vi "Actor Core.vi"(8 "error in":errorcluster, 11 "DAQ in":refnum<class "DAQ.lvclass">) -> (0 "error out":errorcluster, 3 "Actor out":refnum<class "Actor.lvclass">)   [LabVIEW 2011, in "DAQ.lvclass"]
doc: "(<B>Filename</B>: Actor Framework.lvlib:Actor.lvclass:Actor Core.vi)\n\nReceives messages to the actor, reacts to them, and initiates any error handling that may shut the actor down.\n\nDescendant classes may override this VI to append parallel tasks for the actor to complete while it handles messages. Overrides use the Call Parent Method node."
uses:
  DAQ.lvclass
  <userlib>/_Frameworks/ActorFramework/Actor/Actor.lvclass
  <userlib>/_Frameworks/ActorFramework/Actor/Actor.lvclass/Actor.ctl
  <userlib>/_Frameworks/ActorFramework/Message Enqueuer/Message Enqueuer.lvclass/Message Enqueuer.ctl
  Messages/AcquireData/AcquireData.lvclass
  <userlib>/_Frameworks/ActorFramework/Message Enqueuer/Init from Existing Queue.vi
  <userlib>/_Frameworks/ActorFramework/Message Enqueuer/Message Enqueuer.lvclass
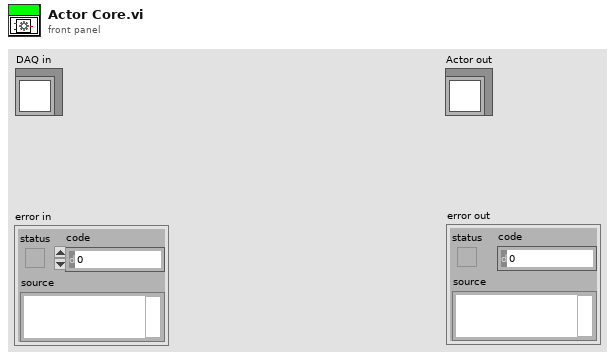
[diagram p1: front panel]
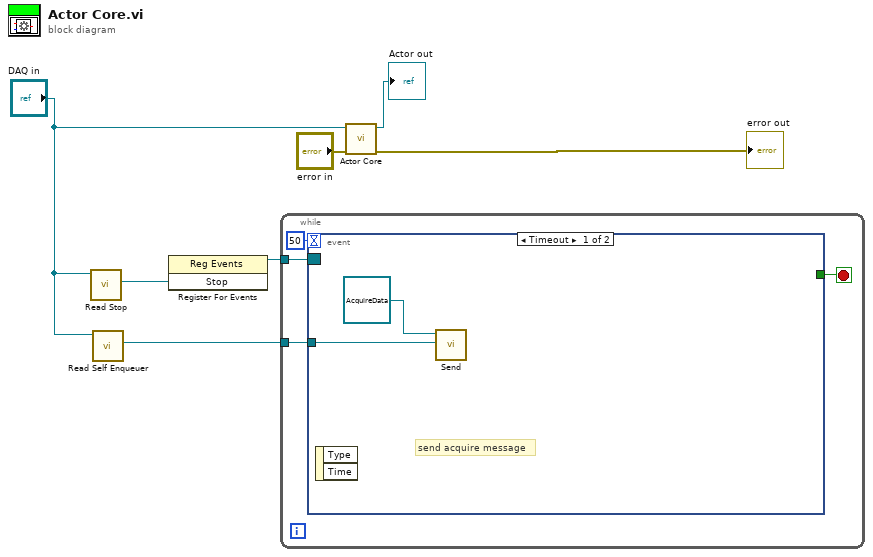
[diagram p0: block diagram]
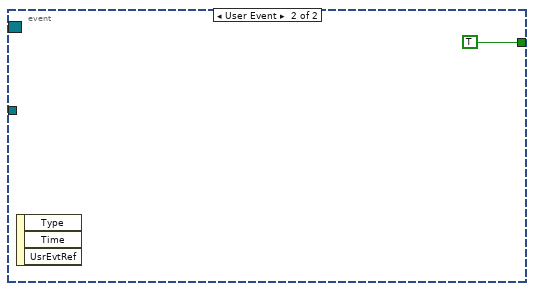
[diagram p2: hidden frame]
diagram:
  n1 = call "Read Stop.vi"("DAQ in"="DAQ in") -> ("Stop"=w3:refnum<user-event>)  [unwired: 9 in, 1 out]
  n2 = call <userlib>:"Read Self Enqueuer.vi"("Actor"="DAQ in") -> ("Self Enqueuer"=w1:refnum<class "Message Enqueuer.lvclass">)  [unwired: 10 in]
  n3 = register-events(w3) -> (reference out=w4:refnum<event-registration>)  [unwired: 2 in, 1 out]
  n4 = while {
    tunnel: w4 -> [w11]
    tunnel: w1 -> [w9]
    stop <- w10 stop-if-true
    n5 = event shown="[0] Timeout" {
      selector: w11 -> [_ _]
      dyn-events: _ -> [_ _]
      timeout: 50 -> [_ _]
      tunnel: [_ TRUE] -> w10
      tunnel: w9 -> [w13 _]
      event Timeout {
        # "send acquire message"
        n6 = event-data() -> ()  [unwired: 1 in, 2 out]
        n7 = call "Send.vi"("Queue"=w13, "AcquireData in"=refnum<class "AcquireData.lvclass"> refnum) -> ()  [unwired: 8 in, 2 out]
      }
      event User Event {
        n8 = event-data() -> ()  [unwired: 1 in, 3 out]
      }
    }
  }
  n9 = call-parent "Actor Core.vi"("error in"="error in", "Actor in"="DAQ in") -> ("error out"=→"error out":errorcluster, "Actor out"=→"Actor out":refnum<class "Actor.lvclass">)  [unwired: 8 in]
